vi "Actor Core.vi"(8 "error in":errorcluster, 11 "Guardian in":refnum<class "Guardian.lvclass">) -> (0 "error out":errorcluster, 3 "Actor out":refnum<class "Actor.lvclass">)   [LabVIEW 2026, in "TALOS.lvlib" / "Guardian.lvlib" / "Guardian.lvclass"]
doc: "(<B>Filename</B>: Actor Framework.lvlib:Actor.lvclass:Actor Core.vi)\n\nReceives messages to the actor, reacts to them, and initiates any error handling that may shut the actor down.\n\nDescendant classes may override this VI to append parallel tasks for the actor to complete while it handles messages. Overrides use the Call Parent Class Method node."
uses:
  Guardian.lvclass
  C:/LabVIEW Code/TALOS/builds/Actor Framework PPL/Actor Framework.lvlibp/1abvi3w/vi.lib/ActorFramework/Actor/Actor.lvclass
  builds/Actor Framework PPL/Actor Framework.lvlibp/1abvi3w/vi.lib/ActorFramework/Actor/Actor.lvclass
  Guardian.lvclass/Guardian.ctl
  Ancestor/Ancestor/Ancestor.lvclass/Ancestor.ctl
  builds/Actor Framework PPL/Actor Framework.lvlibp/1abvi3w/vi.lib/ActorFramework/Message Enqueuer/Message Priority.ctl
  Ancestor/Ancestor Messages/Process EH Error Msg/Process EH Error Msg.lvclass/Process EH Error Msg.ctl
  Support VIs/Generate Error.vi
  FGV/Error Memory/Get Error Description.vi
  Support VIs/Get PC name.vi
  Ancestor/Ancestor/Read ID.vi
  Support VIs/Get Class Name.vi
  <vilib>/Utility/error.llb/Clear Errors.vi
  FGV/Error Memory/Error Memory Core.vi
  <vilib>/AdvancedString/Delimited String to 1D String Array.vi
  <vilib>/AdvancedString/Delimited String to 1D String Array (string).vi
  Support VIs/Circus Root Path.vi
  FGV/Error Memory/Error Crt Lvl checker.vi
  FGV/Error Memory/Error Memory Core.vi/40c8088d-b597-4017-91af-faa98e00292e.vi
  FGV/Error Memory/Error Memory Core.vi/d4a3ab98-063c-4e44-b43d-fbdcfe6c2be2.vi
  builds/Actor Framework PPL/Actor Framework.lvlibp/1abvi3w/vi.lib/ActorFramework/Message Enqueuer/Enqueue.vi
  Support VIs/Global Memory.vi
  <vilib>/Utility/LVClass/Get LV Class Name.vi
  Support VIs/Is in Packed Library.vi
  Support VIs/TALOS Root path.vi
  Support VIs/Read CSV worksheet.vi
  Support VIs/Global Constants.vi
  <vilib>/Utility/error.llb/General Error Handler.vi
  Support VIs/Error Log.vi
  Ancestor/Ancestor/Ancestor.lvclass
  Guardian Messages/I am alive Msg/I am alive Msg.lvclass
  <vilib>/Comparison/Equal/Equal Functor/Equal Functor.lvclass
  Ancestor/Ancestor Messages/Process EH Error Msg/Process EH Error Msg.lvclass
  builds/Actor Framework PPL/Actor Framework.lvlibp/1abvi3w/vi.lib/ActorFramework/Message Enqueuer/Message Enqueuer.lvclass
  TALOS.lvlib
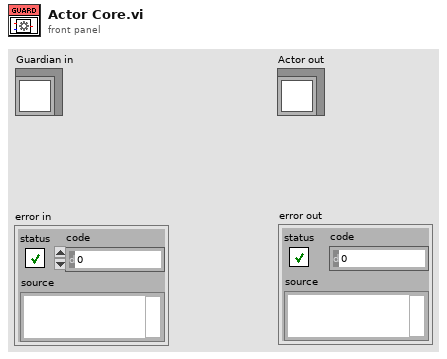
[diagram p1: front panel]
types:
  T1 = cluster{"Stop Helper Loop":refnum<user-event>, "Helper Loop Msg":refnum<user-event>}
  T2 = typedef "Actor Framework.lvlibp/Message Enqueuer.lvclass/Message Priority.ctl" = enum16{"Low", "Normal", "High"}
  T3 = typedef "TALOS.lvlib/Guardian.lvlib/Guardian.lvclass/Helper Loop Msg Selector.ctl" = enum16{"Test String"}
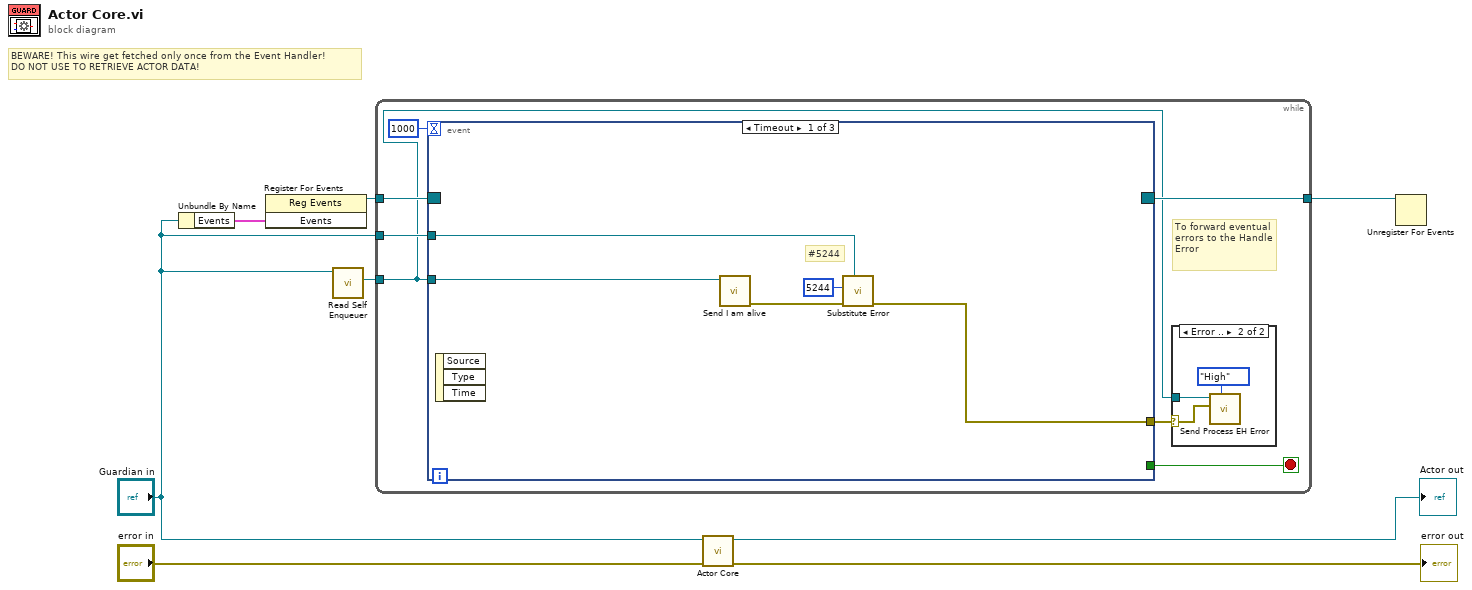
[diagram p0: block diagram]
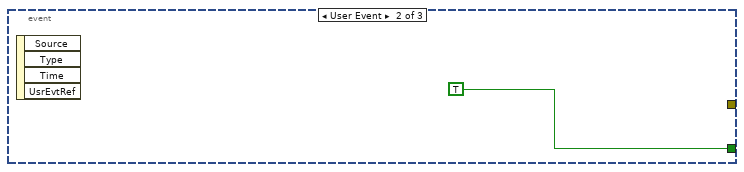
[diagram p2: hidden frame]
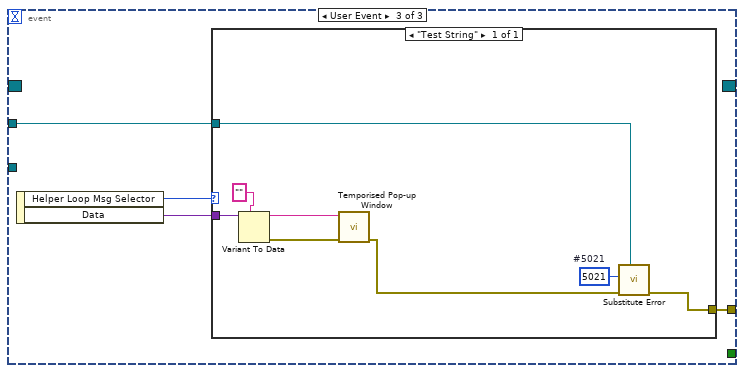
[diagram p3: hidden frame]
diagram:
  # "BEWARE! This wire get fetched only once from the Event Handler!\nDO NOT USE TO RETRIEVE ACTOR DATA!"
  n1 = Unbundle By Name("Guardian in") -> ("Events"=w5:T1)
  n2 = register-events(w5) -> (reference out=w4:refnum<event-registration>)  [unwired: 2 in, 1 out]
  n3 = call "Read Self Enqueuer.vi"("Actor"="Guardian in") -> ("Self Enqueuer"=w6:refnum<class "Message Enqueuer.lvclass">)  [unwired: 10 in]
  n4 = while {
    tunnel: w6 -> [w10]
    tunnel: w4 -> [w15]
    tunnel: [w13] -> w3
    tunnel: "Guardian in" -> [w11]
    stop <- w14 stop-if-true
    # "To forward eventual errors to the Handle Error"
    n5 = event shown="[0] Timeout" {
      selector: w15 -> [_ _ _]
      dyn-events: [_ _ _] -> w13
      timeout: 1000 -> [_ _ _]
      tunnel: w10 -> [w20 _ _]
      tunnel: [_ TRUE _] -> w14
      tunnel: w11 -> [w17 _ w22]
      tunnel: [w18 _ w23] -> w9
      event Timeout {
        # "#5244"
        n6 = event-data() -> ()  [unwired: 1 in, 3 out]
        n7 = call "Send I am alive.vi"("Message Enqueuer"=w20) -> ("error out"=w19:errorcluster)  [unwired: 9 in, 1 out]
        n8 = call "Substitute Error.vi"("LabVIEW Object"=w17, "error in (no error)"=w19, "Error Code"=5244) -> ("error out"=w18:errorcluster)  [unwired: 8 in]
      }
      event User Event {
        n9 = event-data() -> ()  [unwired: 1 in, 4 out]
      }
      event User Event {
        n10 = event-data() -> ("Helper Loop Msg Selector"=w25:T3, "Data"=w24:variant)  [unwired: 1 in]
        n11 = case shown="\"Test String\"" w25 {
          tunnel: w24 -> [w33]
          tunnel: [w26] -> w23
          tunnel: w22 -> [w30]
          frame "Test String" {
            w31 = 5021  # #5021
            n12 = Variant To Data(type="", Variant=w33) -> (data=w28:string, error out=w29:errorcluster)  [unwired: 1 in]
            n13 = call "Temporised Pop-up Window.vi"("error in (no error)"=w29, "Text"=w28) -> ("error out"=w27:errorcluster)  [unwired: 9 in]
            n14 = call "Substitute Error.vi"("LabVIEW Object"=w30, "error in (no error)"=w27, "Error Code"=w31) -> ("error out"=w26:errorcluster)  [unwired: 8 in]
          }
        }
      }
    }
    n15 = case shown="Error .." w9 {
      selector: w9 -> [_ w35]
      tunnel: w10 -> [_ w36]
      frame No Error {
      }
      frame Error {
        n16 = call "Send Process EH Error.vi"("Message Priority (Normal)"=Message_Priority."High", "Error to process"=w35, "Message Enqueuer"=w36) -> ()  [unwired: 7 in, 2 out]
      }
    }
  }
  n17 = call-parent "Actor Core.vi"("error in"="error in", "Actor in"="Guardian in") -> ("error out"=→"error out":errorcluster, "Actor out"=→"Actor out":refnum<class "Actor.lvclass">)  [unwired: 8 in]
  n18 = Unregister For Events(event registration refnum=w3) -> ()  [unwired: 1 in, 1 out]
